vi "IDS_system_getSystemError.vi"(0 "deviceHandle":i32, 3 "error in (no error)":errorcluster) -> (7 "deviceHandle out":i32, 8 "error":i64, 10 "error out":errorcluster)   [LabVIEW 2016]
doc: "int IDS_DLL IDS_system_getSystemError(int64_t * error);"
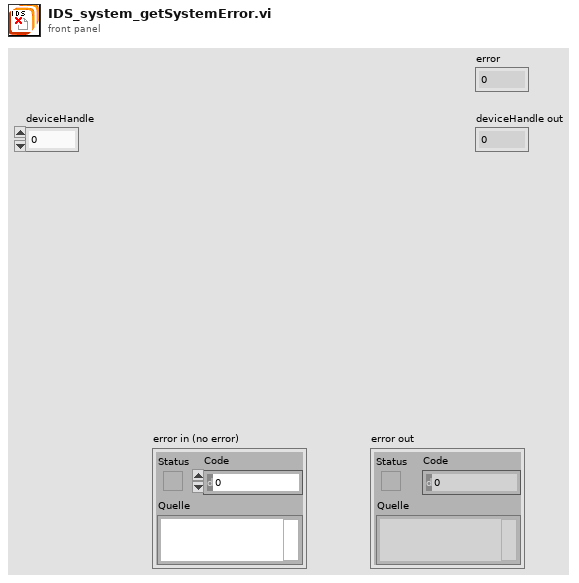
[diagram p1: front panel]
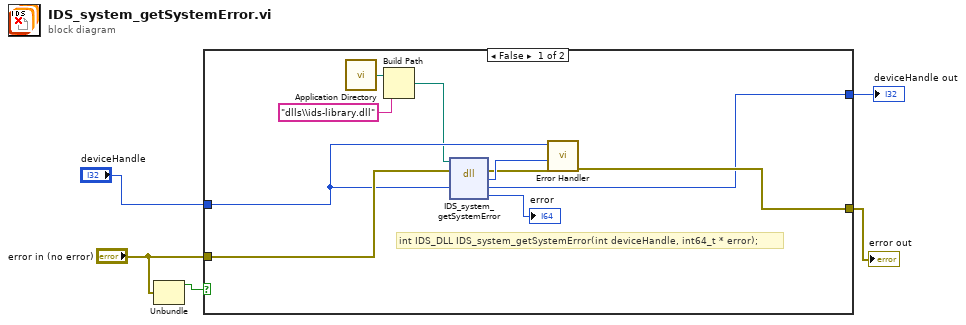
[diagram p0: block diagram]
diagram:
  n1 = Unbundle("error in (no error)") -> ("status"=w3:bool)  [unwired: 2 out]
  n2 = case shown="False" w3 {
    tunnel: "deviceHandle" -> [w11 w17]
    tunnel: "error in (no error)" -> [w12 w16]
    tunnel: [w13 w16] -> w2
    tunnel: [w10 w17] -> w1
    frame False {
      # "int IDS_DLL IDS_system_getSystemError(int deviceHandle, int64_t * error);"
      n3 = call <vilib>:"Application Directory.vi"() -> ("Application Directory"=w8:path)
      n4 = Build Path(base path=w8, name or relative path="dlls\\ids-library.dll" ("ipAddress")) -> (appended path=w6:path)
      n5 = dll-call lib="C:/Users/matheus/Desktop/LabVIEW_Draft_V1.6.0/dlls/ids-library.*" fn="IDS_system_getSystemError"(path in=w6, error in=w12, "deviceHandle"=w11) -> (error out=w14:errorcluster, "Rückgabetyp"=w15:i32, "deviceHandle"=w10:i32, "error"=→"error":i64)  [unwired: 2 in, 1 out]
      n6 = call "Error Handler.vi"("error in (no error)"=w14, "error code"=w15, "deviceHandle"=w11) -> ("error out"=w13:errorcluster)  [unwired: 7 in, 1 out]
    }
    frame True {
    }
  }
  "error out" <- w2
  "deviceHandle out" <- w1
